vi "Read Task.vi"(8 "error in (no error)":errorcluster, 11 "Thermometer DAQmx in":refnum<class "Thermometer DAQmx.lvclass">) -> (0 "error out":errorcluster, 2 "Task":refnum<k21>, 3 "Thermometer DAQmx out":refnum<class "Thermometer DAQmx.lvclass">)   [LabVIEW 2023, in "Thermometer.lvlib" / "Thermometer DAQmx.lvlib" / "Thermometer DAQmx.lvclass"]
uses:
  Thermometer DAQmx.lvclass
  Thermometer DAQmx Config/Thermometer DAQmx Config.lvclass
  Thermometer Base/Thermometer Base.lvclass/Thermometer Base.ctl
  Thermometer DAQmx Config/Thermometer DAQmx Config.lvclass/Thermometer DAQmx Config.ctl
  Thermometer Base/Thermometer Base.lvclass
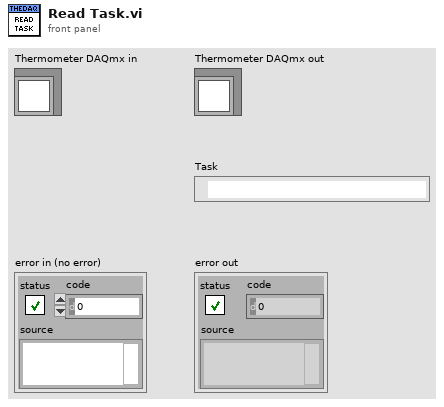
[diagram p1: front panel]
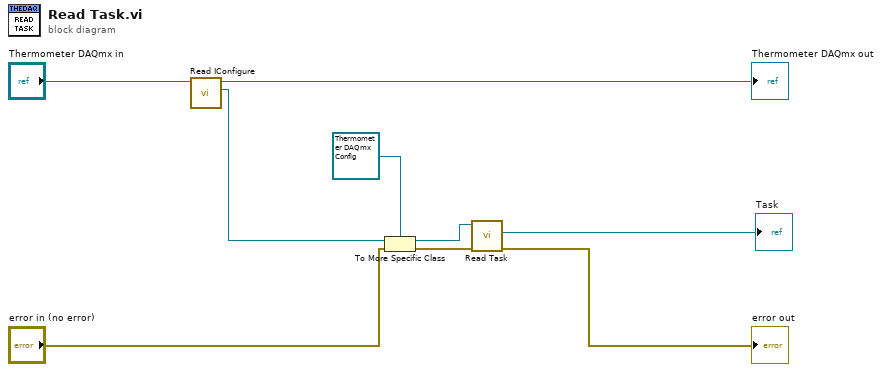
[diagram p0: block diagram]
diagram:
  n1 = call "Read IConfigure.vi"("Thermometer Base in"="Thermometer DAQmx in") -> ("IConfigure"=w4:refnum<class "IConfigure.lvclass">, "Thermometer Base out"=→"Thermometer DAQmx out":refnum<class "Thermometer DAQmx.lvclass">)  [unwired: 8 in, 1 out]
  n2 = To More Specific Class(target class=refnum<class "Thermometer DAQmx Config.lvclass"> refnum ("HAL.lvlib:Thermometer DAQmx.lvlib:Thermometer DAQmx Config.lvclass"), reference=w4, error in="error in (no error)") -> (specific class reference=w6:refnum<class "Thermometer DAQmx Config.lvclass">, error out=w7:errorcluster)
  n3 = call "Read Task.vi"("error in (no error)"=w7, "Thermometer DAQmx Config in"=w6) -> ("error out"=→"error out":errorcluster, "Task"=→"Task":refnum<k21>)  [unwired: 7 in, 1 out]
